vi "Sierra - Frequency Drift test 2-17.vi"() -> ()   [LabVIEW 2015]
doc: "This VI demonstrates a simple procedure for setting up a spectrum analyzer, running an acquisition, and retrieving and plotting the waveform data.\n\nString indicators Binary WF Data and Sgl Float WF Data are initialized to empty strings. Waveform Graph is initialized to 0 for 100000 locations (just an arbitrary number for demonstration purposes).\n\ntkrsa6100 Initialize.vi opens the VISA Resource Name from the information entered by the user. It also presets the instrument by default to the Spectrum measurement. On completion it passes dup VISA Resource Name and error out to the following drivers.\n\nThe next VI to execute is tkrsa6100 Config Frequency.vi. Numeric control Center Freq (MHz)(50) is passed to the VI to set the center frequency to the default 50MHz value. The Set/Read Freq Setting (Set) is not wired since it defaults to SET, which is what is desired in this case. This is the case for all the configuration VI's in the example.\n\nThe next VI to execute is tkrsa6100 Config Spectrum Settings.vi. Enumerated control Spectrum Settings (CENTER FREQUENCY) is passed a Frequency Span constant and numeric control Freq Span (MHz) (40) to set the span to 40MHz.\n\nNext the reference level is set using tkrsa6100 Config RF Input.vi. Enumerated control Input Setting (REFERENCE LEVEL) is passed a Reference Level constant and numeric control Ref Level (dBm)(0) to set the reference level to 0dBm.\n\nNext the acquisition mode is set to single acquisition using tkrsa6100 Config Acquisition.vi. No parameters are passed since the default setting of this VI sets the acquisition mode to single.\n\nA single acquisition is then performed using tkrsa6100 Run Single Acquisition.vi. This VI sends an INIT command followed by a *OPC? Query. When the acquisition is completed the instrument returns a 1 and the next vi executes.\n\nThe binary waveform data is then retrieved by tkrsa6100 Spectrum Msmt Results.vi. The last acquisition data is retrieved by passing constant GET LAST ACQUISITION RESULT to enumerated input Run Acquisition and/or Get Result (RUN ACQUISITION & GET RESULT). The binary data is converted to a comma separated list of single precision floating point numbers by passing constant YES to enumerated input Convert Resp String (NO). The number of display points (total number of data bytes/4) is passed to a Spectral Display property node to scale the x axis of the graph. The binary data string from output Measurement Response String is copied to string indicator Binary WF Data. The converted binary data from output Converted Sgl Float Response String is copied to string indicator Sgl Float WF Data.\n\nSgl Float WF Data is then converted to an array by function Spreadsheet String to Array using a comma as the data separator. The output array is then passed to waveform graph Spectral Display for viewing.\n\nThe VISA Resource Name is closed using tkrsa6100 Close.vi."
panel:
  out "Marker\nResponse String 2":string
  out "Marker\nResponse String":string
  in  "Trig Level (dBm)":dbl=-10.0 min=-170.0 max=50.0 step=0.1
  in  "Ref Level (dBm)(0)":dbl min=-170.0 max=50.0 step=0.1
  in  "Msmt Freq (MHz)":dbl=1000.0 min=0.009 max=20000.0 step=1e-06 format="%.6f"
  in  "VISA Resource Name":refnum<visa-resource-name>
  out "Sgl Float WF Data":string
  out "Binary WF Data":string
  out "Spectral Display":dbl[](graph)
  out "error out":errorcluster {"code" format="%#.0f"}
  # "RSA6106A/6114A Acquire and Fetch\nSpectral Analysis Display"
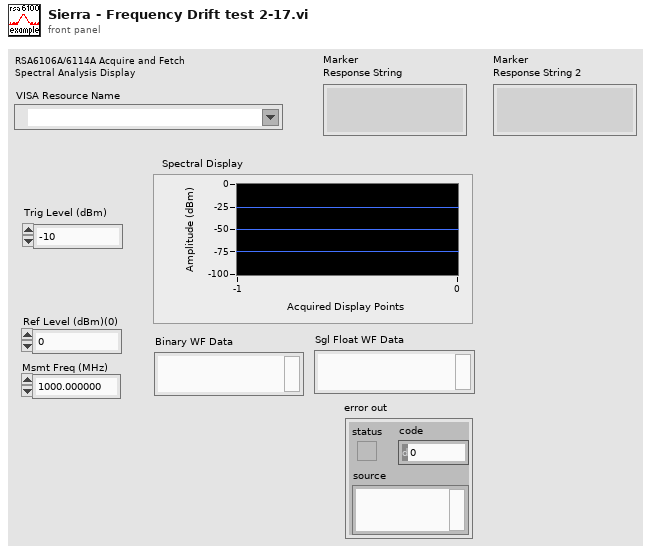
[diagram p1: front panel]
types:
  T1 = enum16{"CENTER FREQUENCY", "FREQUENCY SPAN", "RESOLUTION BW", "MAX REAL TIME SPAN (SET)", "START FREQUENCY", "STOP FREQUENCY", "FREQ STEP SIZE", "AUTO FREQ STEP ON", "AUTO FREQ STEP OFF", "AUTO RES BW ON", "AUTO RES BW OFF", "FFT WINDOW TYPE", "# POINTS", "RBW PROCESS ON", "RBW PROCESS OFF", "GAIN/BW OPTIMIZATION"}
  T2 = enum16{"ANALYSIS REFERENCE", "ANALYSIS LENGTH", "ACTUAL ANALYSIS LENGTH (READ)", "AUTO ANALYSIS LENGTH ON", "AUTO ANALYSIS LENGTH OFF", "ANALYSIS OFFSET", "AUTO ANALYSIS OFFSET ON", "AUTO ANALYSIS OFFSET OFF", "SPECTRUM LENGTH", "ACTUAL SPECTRUM LENGTH (READ)", "AUTO SPECTRUM LENGTH ON", "AUTO SPECTRUM LENGTH OFF", "SPECTRUM OFFSET", "SPECTRUM TIME MODE", "DITHER MODE", "DITHER HW STATUS (READ)", "AUTO SPECTRUM OFFSETS AND ANALYSIS"}
  T3 = enum16{"TRIGGER SOURCE", "TRIGGER ON", "TRIGGER OFF", "TIME DELAY", "TIME POSITION", "TRIGGER EACH SEGMENT ON", "TRIGGER EACH SEGMENT OFF", "TRIGGER TYPE POWER", "TRIGGER TYPE FREQ MASK", "TRIGGER LEVEL", "TRIGGER SLOPE RISING", "TRIGGER SLOPE FALLING", "TDBW MODE ON", "TDBW MODE OFF", "TDBW", "ACTUAL TDBW (READ)", "CREATE NEW FMT (SET)", "SAVE FMT (SET)", "LOAD FMT (SET)", "FMT VIOLATION LOGIC", "FMT RBW AUTO", "FMT RBW MANUAL", "FMT RBW", "FORCE TRIGGER", "Trigger Position Auto"}
  T4 = enum16{"RUN ACQUISITION & GET RESULT", "GET LAST ACQUISITION RESULT"}
  T5 = enum16{"PEAK FIND (SET)", "NEXT PEAK LOWER (SET)", "NEXT PEAK HIGHER (SET)", "NEXT PEAK LEFT (SET)", "NEXT PEAK RIGHT (SET)", "MARKER TIME", "MARKER FREQUENCY (READ)", "DELTA MARKER TIME (READ)", "DELTA MARKER FREQ (READ)"}
  T6 = enum16{"TRACE FUNCTION", "TRACE DETECTION", "TRACE ON", "TRACE OFF", "FREEZE ON", "FREEZE OFF", "AVERAGE COUNT", "CLEAR TRACE (SET)"}
  T7 = enum16{"AVERAGE", "-PEAK", "+PEAK", "+/-PEAK", "SAMPLE"}
  T8 = enum16{"SPECTRUM ANALYZER", "DPSA", "SPECTROGRAM", "AMPL VS TIME", "FREQ VS TIME", "PHASE VS TIME", "IQ VS TIME", "TIME OVERVIEW"}
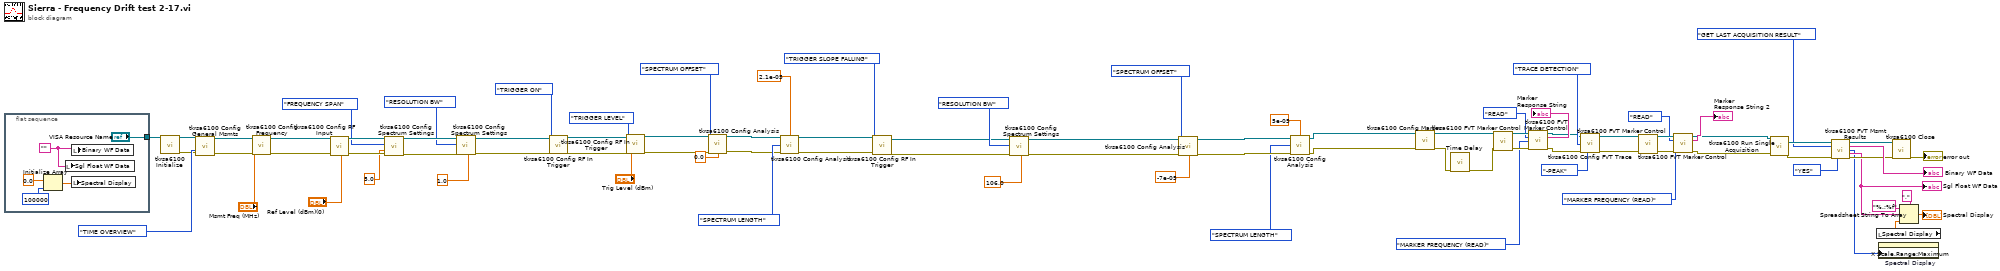
[diagram p0: block diagram]
diagram:
  n1 = flat-sequence {
    tunnel: ["VISA Resource Name"] -> w75
    frame #0 {
      w87 = ""
      n2 = Initialize Array(0.0 ("element"), 100000 ("dimension size")) -> (w89:dbl[])
      n3 = local write "Sgl Float WF Data"(w87) -> ()
      n4 = local write "Spectral Display"(w89) -> ()
      n5 = local write "Binary WF Data"(w87) -> ()
    }
  }
  n6 = call <instrlib>:"tkrsa6100 Initialize.vi"("VISA Resource Name"=w75) -> ("dup VISA Resource Name"=w71:refnum<visa-resource-name>, "error out"=w72:errorcluster)  [unwired: 3 in, 10 out]
  n7 = call <instrlib>:"tkrsa6100 Config General Msmts.vi"("VISA Resource Name"=w71, "Measurement\n(SPECTRUM ANALYZER)"=T8."TIME OVERVIEW" ("Measurement\n(SPECTRUM ANALYZER)"), "error in (no error)"=w72) -> ("dup VISA Resource Name"=w32:refnum<visa-resource-name>, "error out"=w31:errorcluster)  [unwired: 10 in, 1 out]
  n8 = call <instrlib>:"tkrsa6100 Config Frequency.vi"("VISA Resource Name"=w32, "Msmt Freq (MHz)\n(1000)"="Msmt Freq (MHz)", "error in (no error)"=w31) -> ("dup VISA Resource Name"=w30:refnum<visa-resource-name>, "error out"=w29:errorcluster)  [unwired: 1 in, 10 out]
  n9 = call <instrlib>:"tkrsa6100 Config RF Input.vi"("VISA Resource Name"=w30, "Ref Level (0)"="Ref Level (dBm)(0)", "error in (no error)"=w29) -> ("dup VISA Resource Name"=w16:refnum<visa-resource-name>, "error out"=w13:errorcluster)  [unwired: 4 in, 7 out]
  n10 = call <instrlib>:"tkrsa6100 Config Spectrum Settings.vi"("VISA Resource Name"=w16, "Spectrum Settings\n (CENTER FREQUENCY)"=T1."FREQUENCY SPAN" ("Spectrum Settings\n (CENTER FREQUENCY)"), "Freq Span\n(MHz)(40)"=5.0 ("Freq Span\n(MHz)(40)"), "error in (no error)"=w13) -> ("dup VISA Resource Name"=w15:refnum<visa-resource-name>, "error out"=w12:errorcluster)  [unwired: 13 in, 1 out]
  n11 = call <instrlib>:"tkrsa6100 Config Spectrum Settings.vi"("VISA Resource Name"=w15, "Spectrum Settings\n (CENTER FREQUENCY)"=T1."RESOLUTION BW" ("Spectrum Settings\n (CENTER FREQUENCY)"), "error in (no error)"=w12, "Res BW (KHz)\n(300)"=1.0 ("Res BW (KHz)\n(300)")) -> ("dup VISA Resource Name"=w14:refnum<visa-resource-name>, "error out"=w11:errorcluster)  [unwired: 13 in, 1 out]
  n12 = call <instrlib>:"tkrsa6100 Config RF In Trigger.vi"("VISA Resource Name"=w14, "Trigger Settings\n(TRIGGER SOURCE)"=T3."TRIGGER ON" ("Trigger Settings\n(TRIGGER SOURCE)"), "error in (no error)"=w11) -> ("dup VISA Resource Name"=w52:refnum<visa-resource-name>, "error out"=w53:errorcluster)  [unwired: 14 in, 1 out]
  n13 = call <instrlib>:"tkrsa6100 Config RF In Trigger.vi"("VISA Resource Name"=w52, "Trigger Settings\n(TRIGGER SOURCE)"=T3."TRIGGER LEVEL" ("Trigger Settings\n(TRIGGER SOURCE)"), "error in (no error)"=w53, "Trig Level\n(dBm)(-10)"="Trig Level (dBm)") -> ("dup VISA Resource Name"=w51:refnum<visa-resource-name>, "error out"=w28:errorcluster)  [unwired: 13 in, 1 out]
  n14 = call <instrlib>:"tkrsa6100 Config Analysis.vi"("VISA Resource Name"=w51, "Analysis Setting\n(ANALYSIS REFERENCE)"=T2."SPECTRUM OFFSET" ("Analysis Setting\n(ANALYSIS REFERENCE)"), "error in (no error)"=w28, "Offset Tme (S)(0)"=0.0) -> ("dup VISA Resource Name"=w49:refnum<visa-resource-name>, "error out"=w50:errorcluster)  [unwired: 9 in, 1 out]
  n15 = call <instrlib>:"tkrsa6100 Config Analysis.vi"("VISA Resource Name"=w49, "Length (S)(0.022)"=2.1e-05, "Analysis Setting\n(ANALYSIS REFERENCE)"=T2."SPECTRUM LENGTH" ("Analysis Setting\n(ANALYSIS REFERENCE)"), "error in (no error)"=w50) -> ("dup VISA Resource Name"=w24:refnum<visa-resource-name>, "error out"=w23:errorcluster)  [unwired: 9 in, 1 out]
  n16 = call <instrlib>:"tkrsa6100 Config RF In Trigger.vi"("VISA Resource Name"=w24, "Trigger Settings\n(TRIGGER SOURCE)"=T3."TRIGGER SLOPE FALLING" ("Trigger Settings\n(TRIGGER SOURCE)"), "error in (no error)"=w23) -> ("dup VISA Resource Name"=w4:refnum<visa-resource-name>, "error out"=w3:errorcluster)  [unwired: 14 in, 1 out]
  n17 = call <instrlib>:"tkrsa6100 Config Spectrum Settings.vi"("VISA Resource Name"=w4, "Spectrum Settings\n (CENTER FREQUENCY)"=T1."RESOLUTION BW" ("Spectrum Settings\n (CENTER FREQUENCY)"), "error in (no error)"=w3, "Res BW (KHz)\n(300)"=106.0 ("Res BW (KHz)\n(300)")) -> ("dup VISA Resource Name"=w2:refnum<visa-resource-name>, "error out"=w1:errorcluster)  [unwired: 13 in, 1 out]
  n18 = call <instrlib>:"tkrsa6100 Config Analysis.vi"("VISA Resource Name"=w2, "Analysis Setting\n(ANALYSIS REFERENCE)"=T2."SPECTRUM OFFSET" ("Analysis Setting\n(ANALYSIS REFERENCE)"), "error in (no error)"=w1, "Offset Tme (S)(0)"=-7e-05) -> ("dup VISA Resource Name"=w22:refnum<visa-resource-name>, "error out"=w21:errorcluster)  [unwired: 9 in, 1 out]
  n19 = call <instrlib>:"tkrsa6100 Config Analysis.vi"("VISA Resource Name"=w22, "Length (S)(0.022)"=5e-05, "Analysis Setting\n(ANALYSIS REFERENCE)"=T2."SPECTRUM LENGTH" ("Analysis Setting\n(ANALYSIS REFERENCE)"), "error in (no error)"=w21) -> ("dup VISA Resource Name"=w20:refnum<visa-resource-name>, "error out"=w19:errorcluster)  [unwired: 9 in, 1 out]
  n20 = call <instrlib>:"tkrsa6100 Config Marker.vi"("VISA Resource Name"=w20, "error in (no error)"=w19) -> ("dup VISA Resource Name"=w63:refnum<visa-resource-name>, "error out"=w58:errorcluster)  [unwired: 11 in, 1 out]
  n21 = call "Time Delay"("error in (no error)"=w58) -> ("error out"=w57:errorcluster)  [unwired: 10 in]
  n22 = call <instrlib>:"tkrsa6100 FVT Marker Control.vi"("VISA Resource Name"=w63, "error in (no error)"=w57) -> ("dup VISA Resource Name"=w62:refnum<visa-resource-name>, "error out"=w61:errorcluster)  [unwired: 11 in, 1 out]
  n23 = call <instrlib>:"tkrsa6100 FVT Marker Control.vi"("VISA Resource Name"=w62, "Set/Read\nMarker Functions (SET)"=enum16{"SET", "READ"}."READ" ("Set/Read\nMarker Functions (SET)"), "Marker Function\n(PEAK FIND)"=T5."MARKER FREQUENCY (READ)" ("Marker Function\n(PEAK FIND)"), "error in (no error)"=w61) -> ("dup VISA Resource Name"=w41:refnum<visa-resource-name>, "Marker\nResponse String"=→"Marker\nResponse String":string, "error out"=w40:errorcluster)  [unwired: 9 in]
  n24 = call <instrlib>:"tkrsa6100 Config FVT Trace.vi"("VISA Resource Name"=w41, "Trace Setting\n(TRACE FUNCTION)"=T6."TRACE DETECTION" ("Trace Setting\n(TRACE FUNCTION)"), "error in (no error)"=w40, "Trace Detection\n(AVERAGE)"=T7."-PEAK" ("Trace Detection\n(AVERAGE)")) -> ("dup VISA Resource Name"=w39:refnum<visa-resource-name>, "error out"=w38:errorcluster)  [unwired: 9 in, 1 out]
  n25 = call <instrlib>:"tkrsa6100 FVT Marker Control.vi"("VISA Resource Name"=w39, "error in (no error)"=w38) -> ("dup VISA Resource Name"=w44:refnum<visa-resource-name>, "error out"=w43:errorcluster)  [unwired: 11 in, 1 out]
  n26 = call <instrlib>:"tkrsa6100 FVT Marker Control.vi"("VISA Resource Name"=w44, "Set/Read\nMarker Functions (SET)"=enum16{"SET", "READ"}."READ" ("Set/Read\nMarker Functions (SET)"), "Marker Function\n(PEAK FIND)"=T5."MARKER FREQUENCY (READ)" ("Marker Function\n(PEAK FIND)"), "error in (no error)"=w43) -> ("dup VISA Resource Name"=w34:refnum<visa-resource-name>, "Marker\nResponse String"=→"Marker\nResponse String 2":string, "error out"=w35:errorcluster)  [unwired: 9 in]
  n27 = call <instrlib>:"tkrsa6100 Run Single Acquisition.vi"("VISA Resource Name"=w34, "error in (no error)"=w35) -> ("dup VISA Resource Name"=w56:refnum<visa-resource-name>, "error out"=w55:errorcluster)  [unwired: 12 out]
  n28 = call <instrlib>:"tkrsa6100 FVT Msmt Results.vi"("VISA Resource Name"=w56, "Run Acquisition and/or \nGet Result (RUN ACQUISITION & GET RESULT)"=T4."GET LAST ACQUISITION RESULT" ("Run Acquisition and/or \nGet Result (RUN ACQUISITION & GET RESULT)"), "error in (no error)"=w55, "Convert Resp\nString(NO)"=enum16{"NO", "YES"}."YES" ("Convert Resp\nString(NO)")) -> ("dup VISA Resource Name"=w78:refnum<visa-resource-name>, "Measurement\nResponse String"=→"Binary WF Data":string, "# Data Points"=w76:i32, "Converted Sgl Float\nResponse String"=w77:string, "error out"=w80:errorcluster)  [unwired: 7 in]
  "Sgl Float WF Data" <- w77
  n29 = local read "Spectral Display"() -> (w85:dbl[])
  n30 = property on="Spectral Display" class="WFGraph (strict)"("X Scale.Range:Maximum"=w76) -> ()  [unwired: 2 in, 2 out]
  n31 = call <instrlib>:"tkrsa6100 Close.vi"("VISA Resource Name"=w78, "error in (no error)"=w80) -> ("error out"=→"error out":errorcluster)  [unwired: 13 out]
  n32 = Spreadsheet String To Array(delimiter (Tab)=",", format string="%.;%f", spreadsheet string=w77, array type (2D Dbl)=w85) -> (array=→"Spectral Display":dbl[])
